vi "GenNet Format System Message for MsgQ.vi"(9 "Payload":variant, 10 "Source Name":string, 11 "Identifer":string) -> (2 "System Message Argument":T1, 3 "System Message constant":string)   [LabVIEW 2014, in "hse-gennet.lvlib"]
doc: "Formats the contents of a System Message"
uses:
  hse-gennet.lvlib
  hse-dqmh/Controls/System Message Argument--cluster.ctl
  hse-dqmh/Controls/System Message Source.ctl
  hse-dqmh/hse-dqmh.lvlib
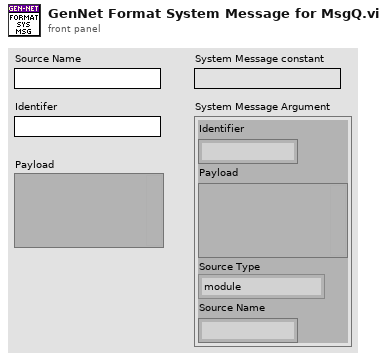
[diagram p1: front panel]
types:
  T1 = typedef "hse-dqmh.lvlib/System Message Argument--cluster.ctl" = cluster{"Identifier":string, "Payload":variant, "Source Type":T2, "Source Name":string}
  T2 = typedef "hse-dqmh.lvlib/System Message Source.ctl" = enum16{"module", "application", "network"}
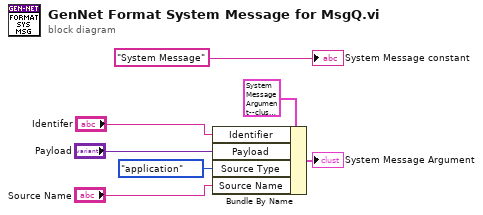
[diagram p0: block diagram]
diagram:
  n1 = Bundle By Name(cluster=T1 {"Identifier"="", "Payload"=variant, "Source Type"=enum."module", "Source Name"=""} ("System Message Argument"), "Identifier"="Identifer", "Payload"="Payload", "Source Type"=System_Message_Source."application" ("System Message Source"), "Source Name"="Source Name") -> (→"System Message Argument":T1)
  "System Message constant" <- "System Message" ("Message")
